vi "amc_Globals.vi"() -> ()   [LabVIEW 2011, in "ART2 Test Panel.lvlib" / "TLB_Dependencies.lvlib"]
uses:
  TLB_Dependencies.lvlib
panel:
  in  "Dispatcher VI Name":string="AMC Dispatcher.vi"
  in  "UDP Port":u16=54321
  in  "Message Dispatch Process Name":string="amcdispatch"
  out "Running":bool
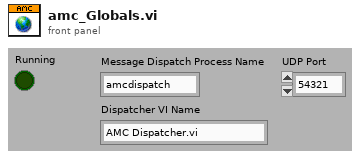
[diagram p1: front panel]
diagram:
